vi "Ex12.vi"() -> ()   [LabVIEW 2016]
uses:
  <vilib>/Analysis/polynomials.llb/Unique Numbers and Multiplicity (DBL).vi
  <vilib>/Analysis/NI_AALPro.lvlib
panel:
  out "중복된 수":dbl[][](array[numeric])
  out "전체 중복 수":dbl[][](array[numeric])
  out "발생":dbl[](array[numeric])
  out "Unique Numbers":dbl[](array[numeric]) caption="중복을 제외한 랜덤 넘버" format="%#.6g"
  out "Sorting":dbl[](array[numeric])
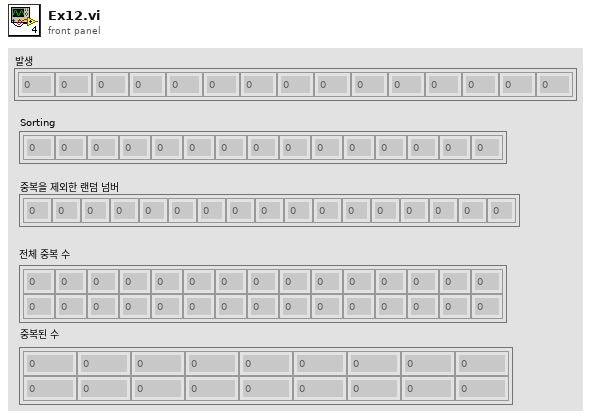
[diagram p1: front panel]
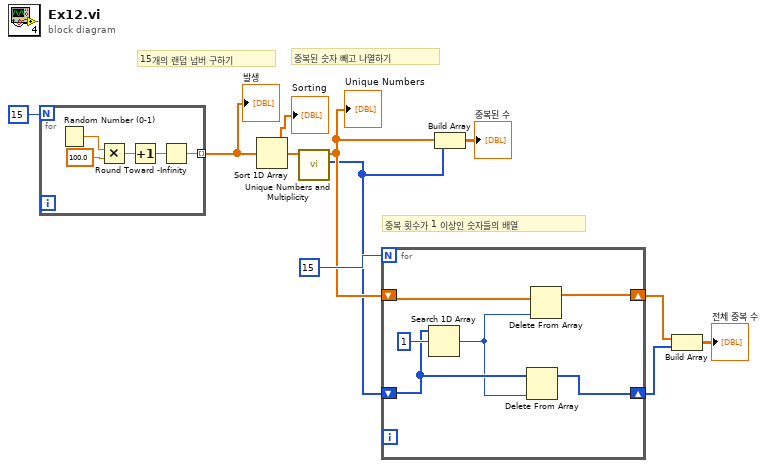
[diagram p0: block diagram]
diagram:
  # "중복 횟수가 1 이상인 숫자들의 배열"
  # "15개의 랜덤 넘버 구하기"
  # "중복된 숫자 빼고 나열하기"
  n1 = for {
    N: 15 -> [_]
    tunnel: [w11] -> w9 mode=indexing
    n2 = Random Number (0-1)() -> (number: 0 to 1=w15:dbl)
    n3 = Multiply(x=w15, y=100.0) -> (x*y=w13:dbl)
    n4 = Increment(x=w13) -> (x+1=w12:dbl)
    n5 = Round Toward -Infinity(1:w12) -> (0:w11:dbl)
  }
  "발생" <- w9
  n6 = Sort 1D Array(array=w9) -> (sorted array=w8:dbl[])
  "Sorting" <- w8
  n7 = call-poly <vilib>:"Unique Numbers and Multiplicity.vi"("Numbers"=w8) -> ("Multiplicity"=w2:u32[], "Unique Numbers"=w3:dbl[])  [unwired: 8 in, 1 out]
  "Unique Numbers" <- w3
  n8 = for {
    N: 15 -> [_]
    shift-right: [w16] -> w5
    shift-left: w2 -> [w18]
    shift-right: [w19] -> w6
    shift-left: w3 -> [w20]
    n9 = Search 1D Array(1D array=w18, element=1 ("시작 인덱스(0)")) -> (index of element=w17:i32)  [unwired: 1 in]
    n10 = Delete From Array(array=w18, index=w17) -> (array with subset deleted=w16:u32[])  [unwired: 1 in, 1 out]
    n11 = Delete From Array(array=w20, index=w17) -> (array with subset deleted=w19:dbl[])  [unwired: 1 in, 1 out]
  }
  n12 = Build Array(w3, w2) -> (→"중복된 수":dbl[][])
  n13 = Build Array(w6, w5) -> (→"전체 중복 수":dbl[][])
